vi "Read Measurement Counts.vi"(8 "error in (no error)":errorcluster, 11 "VISA resource name":refnum<visa-resource-name>) -> (0 "error out":errorcluster, 2 "Data Points":i32, 3 "VISA resource name out":refnum<visa-resource-name>)   [LabVIEW 2020, in "Agilent 3446X Series.lvlib"]
doc: "Returns the total number of measurements currently in reading memory."
uses:
  <instrlib>/Agilent 3446X Series/Agilent 3446X Series.lvlib
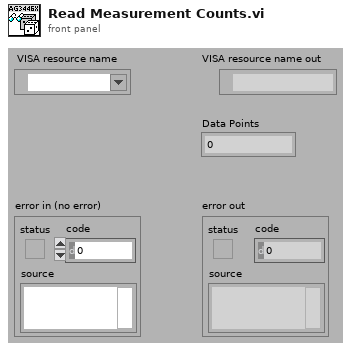
[diagram p1: front panel]
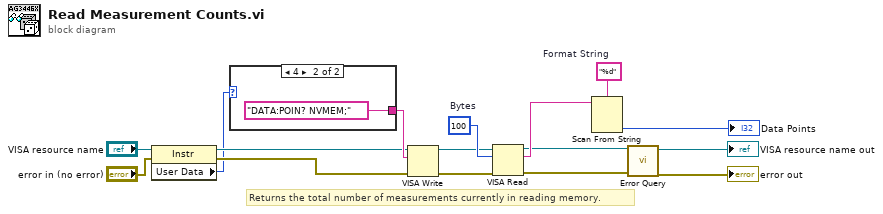
[diagram p0: block diagram]
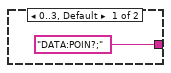
[diagram p2: hidden frame]
diagram:
  w12 = "%d"  # Format String
  w13 = u32 100  # Bytes
  # "Returns the total number of measurements currently in reading memory."
  n1 = property class="Instr"(reference="VISA resource name", error in="error in (no error)") -> (reference out=w4:refnum<visa-resource-name>, error out=w2:errorcluster, "User Data"=w1:u32)
  n2 = case shown="4" w1 {
    tunnel: ["DATA:POIN?;" "DATA:POIN? NVMEM;"] -> w16
    frame 0..3, Default {
    }
    frame 4 {
    }
  }
  n3 = VISA Write(VISA resource name=w4, write buffer=w16, error in (no error)=w2) -> (VISA resource name out=w10:refnum<visa-resource-name>, error out=w9:errorcluster)  [unwired: 1 out]
  n4 = VISA Read(VISA resource name=w10, byte count=w13, error in (no error)=w9) -> (VISA resource name out=w8:refnum<visa-resource-name>, read buffer=w11:string, error out=w7:errorcluster)  [unwired: 1 out]
  n5 = Scan From String(format string=w12, input string=w11) -> (output 1=→"Data Points":i32)  [unwired: 2 in, 4 out]
  n6 = call <instrlib>:"Error Query.vi"("error in (no error)"=w7, "VISA resource name"=w8) -> ("error out"=→"error out":errorcluster, "VISA resource name out"=→"VISA resource name out":refnum<visa-resource-name>)  [unwired: 8 out]
